vi "stop.vi"(8 "error in (no error)":errorcluster, 11 "Simple Sequencer API in":refnum<class "Simple Sequencer API.lvclass">) -> (0 "error out":errorcluster, 3 "Simple Sequencer API out":refnum<class "Simple Sequencer API.lvclass">)   [LabVIEW 2015, in "Simple Sequencer API.lvclass"]
doc: "Stops the execution of the configured sequences after the next sequence completes. For safety reasons, individual sequences cannot be aborted. Once stopped, the sequences cannot be resumed. Instead a new call must be made to 'run sequences'."
uses:
  Simple Sequencer API.lvclass
  module/execution/sequencer commands.ctl
  Simple Sequencer API.lvclass/Simple Sequencer API.ctl
  <vilib>/NI/AMC/Create Single Message.vi
  <vilib>/NI/AMC/Update Message Routing Info.vi
  <vilib>/NI/AMC/Send Message.vi
  <vilib>/NI/AMC/AMC.lvlib
  module/execution/Simple Sequencer TBM runtime.lvclass
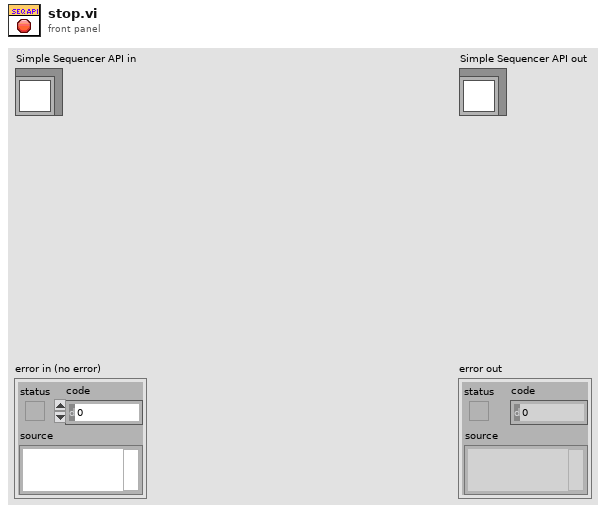
[diagram p1: front panel]
types:
  T1 = typedef "Simple Sequencer TBM runtime.lvclass/sequencer commands.ctl" = enum16{"Run", "Pause", "Resume", "Stop"}
  T2 = typedef "AMC.lvlib/Message Queue.ctl" = refnum<queue>
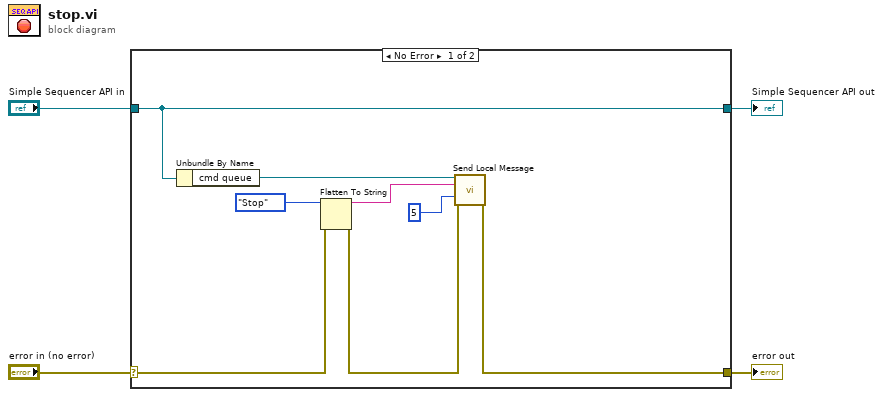
[diagram p0: block diagram]
diagram:
  n1 = case shown="No Error" "error in (no error)" {
    selector: "error in (no error)" -> [w7 w14]
    tunnel: [w5 w14] -> w3
    tunnel: [w8 w13] -> w1
    tunnel: "Simple Sequencer API in" -> [w8 w13]
    frame No Error {
      n2 = Unbundle By Name(w8) -> ("cmd queue"=w12:T2)
      n3 = Flatten To String(anything=sequencer_commands."Stop" ("Commands"), error in (no error)=w7) -> (data string=w9:string, error out=w6:errorcluster)  [unwired: 2 in, 1 out]
      n4 = call <vilib>:"Send Local Message.vi"("message queue in"=w12, "message name"=w9, "timeout (-1 ms)"=5, "error in"=w6) -> ("error out"=w5:errorcluster)  [unwired: 9 in, 2 out]
    }
    frame Error {
    }
  }
  "error out" <- w3
  "Simple Sequencer API out" <- w1
